vi "Main.vi"(7 "sweep rate, /min":dbl=0.2, 8 "sweep to:":dbl=4.0, 9 "sweep":T8(radio)=enum."2636a_smub") -> ()   [LabVIEW 2021] (continued)
                              }
                              frame True {
                                # "we are  measuring voltage on 2636A smua (2636A_smua_v)"
                                n1007 = local read "2614A addr"() -> (w1225:refnum<visa-resource-name>)
                                n1008 = call "SinglePointMeasurement.vi"("Measure"=Measure."Voltage", "Channel"=Channel."a", "VISA resource name 2"=w1225) -> ("Measuremet"=w1227:dbl)  [unwired: 3 in, 4 out]
                                n1009 = Build Array (concatenate)(w1230, w1227) -> (w1229:dbl[])
                              }
                            }
                            n1010 = property on="data" class="Arr (strict)"("Value"=w1223) -> ()  [unwired: 2 in, 2 out]
                          }
                          frame #25 {
                            # "check if current on\nKeithley 2636A smua\nis to be measured"
                            n1011 = local read "2636A smua meas i"() -> (w1231:bool)
                            n1012 = property on="data" class="Arr (strict)"() -> ("Value"=w1232:dbl[])  [unwired: 2 in, 2 out]
                            n1013 = case shown="True" w1231 {
                              tunnel: w1232 -> [w1234 w1237]
                              tunnel: [w1234 w1236] -> w1233
                              frame False {
                                # "we are not measuring current on 2636A smua (2636A_smua_i)"
                              }
                              frame True {
                                # "we are  measuring current on 2636A smua (2636A_smua_i)"
                                n1014 = stacked-sequence {
                                tunnel: [_ w1246] -> w1235
                                frame #0 {
                                n1015 = local read "auto\nrange A"() -> (w1241:bool)
                                n1016 = local read "2614A addr"() -> (w1244:refnum<visa-resource-name>)
                                n1017 = Select(t="smua.AUTORANGE_ON", s=w1241, f="smua.AUTORANGE_OFF") -> (s? t:f=w1239:string)
                                n1018 = Concatenate Strings("smua.measure.autorangei = ", w1239) -> (w1238:string)
                                n1019 = VISA Write(VISA resource name=w1244, write buffer=w1238) -> ()  [unwired: 1 in, 3 out]
                                }
                                frame #1 {
                                n1020 = local read "2614A addr"() -> (w1248:refnum<visa-resource-name>)
                                n1021 = call "SinglePointMeasurement.vi"("Measure"=Measure."Current", "Channel"=Channel."a", "VISA resource name 2"=w1248) -> ("Measuremet"=w1246:dbl)  [unwired: 3 in, 4 out]
                                }
                                }
                                n1022 = Build Array (concatenate)(w1237, w1235) -> (w1236:dbl[])
                              }
                            }
                            n1023 = property on="data" class="Arr (strict)"("Value"=w1233) -> ()  [unwired: 2 in, 2 out]
                          }
                          frame #26 {
                            # "check if voltage on\nKeithley 2636A smub\nis to be measured"
                            n1024 = local read "2636A smub meas v"() -> (w1249:bool)
                            n1025 = property on="data" class="Arr (strict)"() -> ("Value"=w1250:dbl[])  [unwired: 2 in, 2 out]
                            n1026 = case shown="True" w1249 {
                              tunnel: w1250 -> [w1252 w1258]
                              tunnel: [w1252 w1257] -> w1251
                              frame False {
                                # "we are not measuring voltage on 2636A smub (2636A_smub_v)"
                              }
                              frame True {
                                # "we are  measuring voltage on 2636A smub (2636A_smub_v)"
                                n1027 = local read "2614A addr"() -> (w1256:refnum<visa-resource-name>)
                                n1028 = call "SinglePointMeasurement.vi"("Measure"=Measure."Voltage", "Channel"=Channel."b", "VISA resource name 2"=w1256) -> ("Measuremet"=w1254:dbl)  [unwired: 3 in, 4 out]
                                n1029 = Build Array (concatenate)(w1258, w1254) -> (w1257:dbl[])
                              }
                            }
                            n1030 = property on="data" class="Arr (strict)"("Value"=w1251) -> ()  [unwired: 2 in, 2 out]
                          }
                          frame #27 {
                            # "check if current on\nKeithley 2636A smub\nis to be measured"
                            n1031 = local read "2636A smub meas i"() -> (w1259:bool)
                            n1032 = property on="data" class="Arr (strict)"() -> ("Value"=w1260:dbl[])  [unwired: 2 in, 2 out]
                            n1033 = case shown="True" w1259 {
                              tunnel: w1260 -> [w1262 w1265]
                              tunnel: [w1262 w1264] -> w1261
                              frame False {
                                # "we are not measuring current on 2636A smub (2636A_smub_i)"
                              }
                              frame True {
                                # "we are  measuring current on 2636A smub (2636A_smub_i)"
                                n1034 = stacked-sequence {
                                tunnel: [_ w1274] -> w1263
                                frame #0 {
                                n1035 = local read "auto\nrange B"() -> (w1269:bool)
                                n1036 = local read "2614A addr"() -> (w1272:refnum<visa-resource-name>)
                                n1037 = Select(t="smub.AUTORANGE_ON", s=w1269, f="smub.AUTORANGE_OFF") -> (s? t:f=w1267:string)
                                n1038 = Concatenate Strings("smub.measure.autorangei = ", w1267) -> (w1266:string)
                                n1039 = VISA Write(VISA resource name=w1272, write buffer=w1266) -> ()  [unwired: 1 in, 3 out]
                                }
                                frame #1 {
                                n1040 = local read "2614A addr"() -> (w1276:refnum<visa-resource-name>)
                                n1041 = call "SinglePointMeasurement.vi"("Measure"=Measure."Current", "Channel"=Channel."b", "VISA resource name 2"=w1276) -> ("Measuremet"=w1274:dbl)  [unwired: 3 in, 4 out]
                                }
                                }
                                n1042 = Build Array (concatenate)(w1265, w1263) -> (w1264:dbl[])
                              }
                            }
                            n1043 = property on="data" class="Arr (strict)"("Value"=w1261) -> ()  [unwired: 2 in, 2 out]
                          }
                          frame #28 {
                            # "check if time\nis to be measured"
                            n1044 = property on="data" class="Arr (strict)"() -> ("Value"=w1278:dbl[])  [unwired: 2 in, 2 out]
                            n1045 = local read "measure time"() -> (w1277:bool)
                            n1046 = case shown="True" w1277 {
                              tunnel: w1278 -> [w1280 w1283]
                              tunnel: [w1280 w1282] -> w1279
                              frame False {
                                # "we are not measuring time"
                              }
                              frame True {
                                # "seconds from the beginning of month"
                                # "we are  measuring time"
                                n1047 = Build Array (concatenate)(w1283, 0) -> (w1282:dbl[])
                              }
                            }
                            n1048 = property on="data" class="Arr (strict)"("Value"=w1279) -> ()  [unwired: 2 in, 2 out]
                          }
                          frame #29 {
                            n1049 = local read "MagnetField"() -> (w1284:bool)
                            n1050 = property on="data" class="Arr (strict)"() -> ("Value"=w1285:dbl[])  [unwired: 2 in, 2 out]
                            n1051 = case shown="True" w1284 {
                              tunnel: w1285 -> [w1287 w1292]
                              tunnel: [w1287 w1291] -> w1286
                              frame False {
                                # "we are not Measuring magnetic field on IPS120-0"
                              }
                              frame True {
                                # "Measure magnetic field on IPS120-0"
                                n1052 = local read "iPS_addr_sweep"() -> (w1290:refnum<visa-resource-name>)
                                n1053 = call "iPSread.vi"("iPSreadCtrl"=iPSreadCtrl."MagnetField", "VISA resource name"=w1290) -> ("number"=w1288:dbl)  [unwired: 6 in, 3 out]
                                n1054 = Build Array (concatenate)(w1292, w1288) -> (w1291:dbl[])
                              }
                            }
                            n1055 = property on="data" class="Arr (strict)"("Value"=w1286) -> ()  [unwired: 2 in, 2 out]
                          }
                          frame #30 {
                            n1056 = property on="data" class="Arr (strict)"() -> ("Value"=w1294:dbl[])  [unwired: 2 in, 2 out]
                            n1057 = property on="Magnet_T" class="Bool (strict)"() -> ("Value"=w1293:bool)  [unwired: 2 in, 2 out]
                            n1058 = case shown="True" w1293 {
                              tunnel: w1294 -> [w1296 w1301]
                              tunnel: [w1296 w1300] -> w1295
                              frame False {
                                # "we are not Measuring magnetic field on IPS120-0"
                              }
                              frame True {
                                # "Measure magnetic field on IPS120-0"
                                n1059 = local read "iPS_addr_sweep"() -> (w1299:refnum<visa-resource-name>)
                                n1060 = call "iPSread.vi"("iPSreadCtrl"=iPSreadCtrl."Magnet Temp", "VISA resource name"=w1299) -> ("number"=w1297:dbl)  [unwired: 6 in, 3 out]
                                n1061 = Build Array (concatenate)(w1301, w1297) -> (w1300:dbl[])
                              }
                            }
                            n1062 = property on="data" class="Arr (strict)"("Value"=w1295) -> ()  [unwired: 2 in, 2 out]
                          }
                          frame #31 {
                            n1063 = property on="PT1" class="Bool (strict)"() -> ("Value"=w1302:bool)  [unwired: 2 in, 2 out]
                            n1064 = property on="data" class="Arr (strict)"() -> ("Value"=w1303:dbl[])  [unwired: 2 in, 2 out]
                            n1065 = case shown="True" w1302 {
                              tunnel: w1303 -> [w1305 w1310]
                              tunnel: [w1305 w1309] -> w1304
                              frame False {
                                # "we are not Measuring magnetic field on IPS120-0"
                              }
                              frame True {
                                # "Measure magnetic field on IPS120-0"
                                n1066 = local read "iPS_addr_sweep"() -> (w1308:refnum<visa-resource-name>)
                                n1067 = call "iPSread.vi"("iPSreadCtrl"=iPSreadCtrl."Switch Heater Temp", "VISA resource name"=w1308) -> ("number"=w1306:dbl)  [unwired: 6 in, 3 out]
                                n1068 = Build Array (concatenate)(w1310, w1306) -> (w1309:dbl[])
                              }
                            }
                            n1069 = property on="data" class="Arr (strict)"("Value"=w1304) -> ()  [unwired: 2 in, 2 out]
                          }
                          frame #32 {
                            # "check if current \non 2461 SouceMeter\nis to be measured"
                            n1070 = property on="data" class="Arr (strict)"() -> ("Value"=w1312:dbl[])  [unwired: 2 in, 2 out]
                            n1071 = property on="MC_RuO2" class="Bool (strict)"() -> ("Value"=w1311:bool)  [unwired: 2 in, 2 out]
                            n1072 = case shown="True" w1311 {
                              tunnel: w1312 -> [w1314 w1319]
                              tunnel: [w1314 w1318] -> w1313
                              frame False {
                                # "we are not measuring 2461, voltage (2461_meas_v)"
                              }
                              frame True {
                                # "we are  measuring  Teslatron_iTC_Temp"
                                n1073 = property on="iPS_addr_sweep" class="VISAName"() -> ("Value"=w1315:refnum<visa-resource-name>)  [unwired: 2 in, 2 out]
                                n1074 = call "iTCread.vi"("VISA resource name"=w1315, "iTCreadCtrl"=iTCreadCtrl."Sample Temp") -> ("number"=w1316:dbl)  [unwired: 5 in, 3 out]
                                n1075 = Build Array (concatenate)(w1319, w1316) -> (w1318:dbl[])
                              }
                            }
                            n1076 = property on="data" class="Arr (strict)"("Value"=w1313) -> ()  [unwired: 2 in, 2 out]
                          }
                          frame #33 {
                            # "check if current \non 2461 SouceMeter\nis to be measured"
                            n1077 = property on="Still" class="Bool (strict)"() -> ("Value"=w1320:bool)  [unwired: 2 in, 2 out]
                            n1078 = property on="data" class="Arr (strict)"() -> ("Value"=w1321:dbl[])  [unwired: 2 in, 2 out]
                            n1079 = case shown="True" w1320 {
                              tunnel: w1321 -> [w1323 w1328]
                              tunnel: [w1323 w1327] -> w1322
                              frame False {
                                # "we are not measuring 2461, voltage (2461_meas_v)"
                              }
                              frame True {
                                # "we are  measuring  Teslatron_iTC_Temp"
                                n1080 = property on="iPS_addr_sweep" class="VISAName"() -> ("Value"=w1324:refnum<visa-resource-name>)  [unwired: 2 in, 2 out]
                                n1081 = call "iTCread.vi"("VISA resource name"=w1324, "iTCreadCtrl"=iTCreadCtrl."VTI Temp") -> ("number"=w1325:dbl)  [unwired: 5 in, 3 out]
                                n1082 = Build Array (concatenate)(w1328, w1325) -> (w1327:dbl[])
                              }
                            }
                            n1083 = property on="data" class="Arr (strict)"("Value"=w1322) -> ()  [unwired: 2 in, 2 out]
                          }
                          frame #34 {
                            # "check if current \non 2461 SouceMeter\nis to be measured"
                            n1084 = property on="Cold_Plate" class="Bool (strict)"() -> ("Value"=w1329:bool)  [unwired: 2 in, 2 out]
                            n1085 = property on="data" class="Arr (strict)"() -> ("Value"=w1330:dbl[])  [unwired: 2 in, 2 out]
                            n1086 = case shown="True" w1329 {
                              tunnel: w1330 -> [w1332 w1337]
                              tunnel: [w1332 w1336] -> w1331
                              frame False {
                                # "we are not measuring 2461, voltage (2461_meas_v)"
                              }
                              frame True {
                                # "we are  measuring  Teslatron_iTC_Temp"
                                n1087 = property on="iPS_addr_sweep" class="VISAName"() -> ("Value"=w1333:refnum<visa-resource-name>)  [unwired: 2 in, 2 out]
                                n1088 = call "iTCread.vi"("VISA resource name"=w1333, "iTCreadCtrl"=iTCreadCtrl."PT1 Temp") -> ("number"=w1334:dbl)  [unwired: 5 in, 3 out]
                                n1089 = Build Array (concatenate)(w1337, w1334) -> (w1336:dbl[])
                              }
                            }
                            n1090 = property on="data" class="Arr (strict)"("Value"=w1331) -> ()  [unwired: 2 in, 2 out]
                          }
                          frame #35 {
                            # "check if current \non 2461 SouceMeter\nis to be measured"
                            n1091 = property on="data" class="Arr (strict)"() -> ("Value"=w1339:dbl[])  [unwired: 2 in, 2 out]
                            n1092 = property on="PT2" class="Bool (strict)"() -> ("Value"=w1338:bool)  [unwired: 2 in, 2 out]
                            n1093 = case shown="True" w1338 {
                              tunnel: w1339 -> [w1341 w1346]
                              tunnel: [w1341 w1345] -> w1340
                              frame False {
                                # "we are not measuring 2461, voltage (2461_meas_v)"
                              }
                              frame True {
                                # "we are  measuring  Teslatron_iTC_Temp"
                                n1094 = property on="iPS_addr_sweep" class="VISAName"() -> ("Value"=w1342:refnum<visa-resource-name>)  [unwired: 2 in, 2 out]
                                n1095 = call "iTCread.vi"("VISA resource name"=w1342, "iTCreadCtrl"=iTCreadCtrl."PT2 Temp") -> ("number"=w1343:dbl)  [unwired: 5 in, 3 out]
                                n1096 = Build Array (concatenate)(w1346, w1343) -> (w1345:dbl[])
                              }
                            }
                            n1097 = property on="data" class="Arr (strict)"("Value"=w1340) -> ()  [unwired: 2 in, 2 out]
                          }
                          frame #36 {
                            # "check if current \non 2461 SouceMeter\nis to be measured"
                            n1098 = property on="data" class="Arr (strict)"() -> ("Value"=w1348:dbl[])  [unwired: 2 in, 2 out]
                            n1099 = property on="MC_Cernox" class="Bool (strict)"() -> ("Value"=w1347:bool)  [unwired: 2 in, 2 out]
                            n1100 = case shown="True" w1347 {
                              tunnel: w1348 -> [w1350 w1355]
                              tunnel: [w1350 w1354] -> w1349
                              frame False {
                                # "we are not measuring 2461, voltage (2461_meas_v)"
                              }
                              frame True {
                                # "we are  measuring  Teslatron_iTC_Temp"
                                n1101 = property on="iPS_addr_sweep" class="VISAName"() -> ("Value"=w1351:refnum<visa-resource-name>)  [unwired: 2 in, 2 out]
                                n1102 = call "iTCread.vi"("VISA resource name"=w1351, "iTCreadCtrl"=iTCreadCtrl."VTI Pressure") -> ("number"=w1352:dbl)  [unwired: 5 in, 3 out]
                                n1103 = Build Array (concatenate)(w1355, w1352) -> (w1354:dbl[])
                              }
                            }
                            n1104 = property on="data" class="Arr (strict)"("Value"=w1349) -> ()  [unwired: 2 in, 2 out]
                          }
                        }
                      }
                    }
                  }
                }
              }
            }
          }
          frame #4 {
            n1105 = Enqueue Element(queue=w1356, element="Idle") -> ()  [unwired: 2 in, 3 out]
            n1106 = Wait (ms)(milliseconds to wait="Refresh Time(ms)") -> ()  [unwired: 1 out]
          }
        }
      }
      frame "Line Traces" {
      }
      frame "Start Sweep" {
        w1362 = dbl[][] []  # emty array for data
        # "0 = SR830_1_ip\n1 = SR830_1_oop\n2 = SR830_2_ip\n3 = SR830_2_oop\n4 = SR830_3_ip\n5 = SR830_3_oop\n6 = SR830_4_ip \n7 = SR830_4_oop \n8 = SR830_5_ip \n9 = SR830_5_oop \n10= 2400_1_v \n11= 2400_1_i \n12 = 2400_2_v\n13 = 2400_2_i \n14 = 2400_3_v \n15 = 2400_3_i \n16 = 2182A_1_ch1 \n17 = 2182A_1_ch2 \n18 = 2182A_2_ch1 \n19 = 2182A_2_ch2\n20 = 2182A_3_ch1 \n21 = 2182A_3_ch2 \n22 = 2182A_4_ch1 \n23 = 2182A_4_ch2 \n24 = 2636A_smua_v \n25 = 2636A_smua_i \n26 = 2636A_smub_v \n27 = 2636A_smub_i \n28 = time\n29 = iPS_Field\n30 = iPS_Magnet_T\n31 = iPS__SH_T\n32 = iTC _sample_T\n33 = iTC _VTI_T\n34 = iTC _PT1_T\n35 = iTC _PT2_T\n36 = iTC _VTI_P\n37 = 2461_meas_v\n38= 2461_meas_i\n39= Step_Value\n40= HyperLoop_Step\n41= SuperHyper_Step\n42 = MFLI_V\n43 = MFLI_I"
        # "initial time in seconds\nfrom the beginning of month"
        n1107 = stacked-sequence {
          tunnel: [_ _ w2342 _ _ _] -> w1359
          frame #0 {
            n1108 = local read "2636A smua meas v"() -> (w1369:bool)
            n1109 = local read "2636A smub meas v"() -> (w1367:bool)
            n1110 = local read "2636A smub meas i"() -> (w1366:bool)
            n1111 = local read "2636A smua meas i"() -> (w1368:bool)
            n1112 = property on="sweep" class="RadioBtnsControl (strict)"() -> ("Value"=w1364:T8)  [unwired: 2 in, 2 out]
            n1113 = Compound Arithmetic op=OR(w1369, w1368, w1367, w1366) -> (w1365:bool)
            n1114 = case shown="\"AuxOut0\"" w1364 {
              frame "2400_1" {
                # "add label for the first column in the datafile"
                n1115 = stacked-sequence {
                  frame #0 {
                    n1116 = property on="data_caption" class="Str"("Value"="") -> ()  [unwired: 2 in, 2 out]
                    n1117 = property on="Figure_axis" class="Arr (strict)"("Value"=string[] [] ("Figure_axis_string")) -> ()  [unwired: 2 in, 2 out]
                  }
                  frame #1 {
                    w1372 = "V_sweep_2400_1" ("V_sweep")
                    n1118 = Concatenate Strings(w1372, "\t") -> (w1374:string)
                    n1119 = Build Array(w1372) -> (w1373:string[])
                    n1120 = property on="data_caption" class="Str"("Value"=w1374) -> ()  [unwired: 2 in, 2 out]
                    n1121 = property on="Figure_axis" class="Arr (strict)"("Value"=w1373) -> ()  [unwired: 2 in, 2 out]
                  }
                }
              }
              frame "2400_2" {
                n1122 = stacked-sequence {
                  frame #0 {
                    n1123 = property on="data_caption" class="Str"("Value"="") -> ()  [unwired: 2 in, 2 out]
                    n1124 = property on="Figure_axis" class="Arr (strict)"("Value"=string[] [] ("Figure_axis_string")) -> ()  [unwired: 2 in, 2 out]
                  }
                  frame #1 {
                    w1378 = "V_sweep_2400_2" ("V_sweep")
                    n1125 = Build Array(w1378) -> (w1379:string[])
                    n1126 = Concatenate Strings(w1378, "\t") -> (w1381:string)
                    n1127 = property on="Figure_axis" class="Arr (strict)"("Value"=w1379) -> ()  [unwired: 2 in, 2 out]
                    n1128 = property on="data_caption" class="Str"("Value"=w1381) -> ()  [unwired: 2 in, 2 out]
                  }
                }
              }
              frame "2400_3" {
                n1129 = stacked-sequence {
                  frame #0 {
                    n1130 = property on="data_caption" class="Str"("Value"="") -> ()  [unwired: 2 in, 2 out]
                    n1131 = property on="Figure_axis" class="Arr (strict)"("Value"=string[] [] ("Figure_axis_string")) -> ()  [unwired: 2 in, 2 out]
                  }
                  frame #1 {
                    w1384 = "V_sweep_2400_3" ("V_sweep")
                    n1132 = Concatenate Strings(w1384, "\t") -> (w1387:string)
                    n1133 = Build Array(w1384) -> (w1385:string[])
                    n1134 = property on="data_caption" class="Str"("Value"=w1387) -> ()  [unwired: 2 in, 2 out]
                    n1135 = property on="Figure_axis" class="Arr (strict)"("Value"=w1385) -> ()  [unwired: 2 in, 2 out]
                  }
                }
              }
              frame "2636a_smua" {
                n1136 = stacked-sequence {
                  frame #0 {
                    n1137 = property on="data_caption" class="Str"("Value"="") -> ()  [unwired: 2 in, 2 out]
                    n1138 = property on="Figure_axis" class="Arr (strict)"("Value"=string[] [] ("Figure_axis_string")) -> ()  [unwired: 2 in, 2 out]
                  }
                  frame #1 {
                    w1390 = "V_sweep_2614a_smua" ("V_sweep")
                    n1139 = Concatenate Strings(w1390, "\t") -> (w1393:string)
                    n1140 = Build Array(w1390) -> (w1391:string[])
                    n1141 = property on="data_caption" class="Str"("Value"=w1393) -> ()  [unwired: 2 in, 2 out]
                    n1142 = property on="Figure_axis" class="Arr (strict)"("Value"=w1391) -> ()  [unwired: 2 in, 2 out]
                  }
                }
              }
              frame "2636a_smub" {
                n1143 = stacked-sequence {
                  frame #0 {
                    n1144 = property on="data_caption" class="Str"("Value"="") -> ()  [unwired: 2 in, 2 out]
                    n1145 = property on="Figure_axis" class="Arr (strict)"("Value"=string[] [] ("Figure_axis_string")) -> ()  [unwired: 2 in, 2 out]
                  }
                  frame #1 {
                    w1396 = "V_sweep_2614a_smub" ("V_sweep")
                    n1146 = Build Array(w1396) -> (w1397:string[])
                    n1147 = Concatenate Strings(w1396, "\t") -> (w1399:string)
                    n1148 = property on="Figure_axis" class="Arr (strict)"("Value"=w1397) -> ()  [unwired: 2 in, 2 out]
                    n1149 = property on="data_caption" class="Str"("Value"=w1399) -> ()  [unwired: 2 in, 2 out]
                  }
                }
              }
              frame "time_sweep", Default {
                n1150 = stacked-sequence {
                  frame #0 {
                    n1151 = property on="data_caption" class="Str"("Value"="") -> ()  [unwired: 2 in, 2 out]
                    n1152 = property on="Figure_axis" class="Arr (strict)"("Value"=string[] [] ("Figure_axis_string")) -> ()  [unwired: 2 in, 2 out]
                  }
                  frame #1 {
                    w1402 = "time_sweep" ("V_sweep")
                    n1153 = Build Array(w1402) -> (w1403:string[])
                    n1154 = Concatenate Strings(w1402, "\t") -> (w1404:string)
                    n1155 = property on="Figure_axis" class="Arr (strict)"("Value"=w1403) -> ()  [unwired: 2 in, 2 out]
                    n1156 = property on="data_caption" class="Str"("Value"=w1404) -> ()  [unwired: 2 in, 2 out]
                  }
                }
              }
              frame "iPS" {
                n1157 = stacked-sequence {
                  frame #0 {
                    n1158 = property on="data_caption" class="Str"("Value"="") -> ()  [unwired: 2 in, 2 out]
                    n1159 = property on="Figure_axis" class="Arr (strict)"("Value"=string[] [] ("Figure_axis_string")) -> ()  [unwired: 2 in, 2 out]
                  }
                  frame #1 {
                    w1408 = "Teslatron_iPS_OutputField" ("V_sweep")
                    n1160 = Build Array(w1408) -> (w1409:string[])
                    n1161 = Concatenate Strings(w1408, "\t") -> (w1411:string)
                    n1162 = property on="Figure_axis" class="Arr (strict)"("Value"=w1409) -> ()  [unwired: 2 in, 2 out]
                    n1163 = property on="data_caption" class="Str"("Value"=w1411) -> ()  [unwired: 2 in, 2 out]
                  }
                }
              }
              frame "iTC" {
                n1164 = stacked-sequence {
                  frame #0 {
                    n1165 = property on="data_caption" class="Str"("Value"="") -> ()  [unwired: 2 in, 2 out]
                    n1166 = property on="Figure_axis" class="Arr (strict)"("Value"=string[] ["", "SR830_1_ip", "SR830_1_oop", "SR830_2_ip", "SR830_2_oop", "2461_meas_v", "2461_meas_i", "2636A_smua_v", "2636A_smua_i", "formula"] ("Figure_axis")) -> ()  [unwired: 2 in, 2 out]
                  }
                  frame #1 {
                    w1416 = "Teslatron_iTC_Temp"
                    n1167 = Build Array(w1416) -> (w1415:string[])
                    n1168 = Concatenate Strings(w1416, "\t") -> (w1414:string)
                    n1169 = property on="data_caption" class="Str"("Value"=w1414) -> ()  [unwired: 2 in, 2 out]
                    n1170 = property on="Figure_axis" class="Arr (strict)"("Value"=w1415) -> ()  [unwired: 2 in, 2 out]
                  }
                }
              }
              frame "2461" {
                n1171 = stacked-sequence {
                  frame #0 {
                    n1172 = property on="data_caption" class="Str"("Value"="") -> ()  [unwired: 2 in, 2 out]
                    n1173 = property on="Figure_axis" class="Arr (strict)"("Value"=string[] ["", "SR830_1_ip", "SR830_1_oop", "SR830_2_ip", "SR830_2_oop", "2461_meas_v", "2461_meas_i", "2636A_smua_v", "2636A_smua_i", "formula"] ("Figure_axis")) -> ()  [unwired: 2 in, 2 out]
                  }
                  frame #1 {
                    w1422 = "I_sweep_2461"
                    n1174 = Build Array(w1422) -> (w1421:string[])
                    n1175 = Concatenate Strings(w1422, "\t") -> (w1420:string)
                    n1176 = property on="data_caption" class="Str"("Value"=w1420) -> ()  [unwired: 2 in, 2 out]
                    n1177 = property on="Figure_axis" class="Arr (strict)"("Value"=w1421) -> ()  [unwired: 2 in, 2 out]
                  }
                }
              }
              frame "AuxOut0" {
                n1178 = stacked-sequence {
                  frame #0 {
                    n1179 = property on="data_caption" class="Str"("Value"="") -> ()  [unwired: 2 in, 2 out]
                    n1180 = property on="Figure_axis" class="Arr (strict)"("Value"=string[] ["", "SR830_1_ip", "SR830_1_oop", "SR830_2_ip", "SR830_2_oop", "2461_meas_v", "2461_meas_i", "2636A_smua_v", "2636A_smua_i", "formula"] ("Figure_axis")) -> ()  [unwired: 2 in, 2 out]
                  }
                  frame #1 {
                    w1428 = "V_Sweep_AuxOut0"
                    n1181 = Build Array(w1428) -> (w1427:string[])
                    n1182 = Concatenate Strings(w1428, "\t") -> (w1426:string)
                    n1183 = property on="data_caption" class="Str"("Value"=w1426) -> ()  [unwired: 2 in, 2 out]
                    n1184 = property on="Figure_axis" class="Arr (strict)"("Value"=w1427) -> ()  [unwired: 2 in, 2 out]
                  }
                }
              }
            }
            n1185 = case shown="True" w1365 {
              frame False {
              }
              frame True {
                # "opens session for 2636a system sourcemeter"
                n1186 = local read "2614A addr"() -> (w1430:refnum<visa-resource-name>)
                n1187 = VISA Open(VISA resource name=w1430) -> ()  [unwired: 4 in, 2 out]
              }
            }
          }
          frame #1 {
            # "0 = SR830_1_ip\n1 = SR830_1_oop\n2 = SR830_2_ip\n3 = SR830_2_oop\n4 = SR830_3_ip\n5 = SR830_3_oop\n6 = SR830_4_ip \n7 = SR830_4_oop \n8 = SR830_5_ip \n9 = SR830_5_oop \n10= 2400_1_v \n11= 2400_1_i \n12 = 2400_2_v\n13 = 2400_2_i \n14 = 2400_3_v \n15 = 2400_3_i \n16 = 2182A_1_ch1 \n17 = 2182A_1_ch2 \n18 = 2182A_2_ch1 \n19 = 2182A_2_ch2\n20 = 2182A_3_ch1 \n21 = 2182A_3_ch2 \n22 = 2182A_4_ch1 \n23 = 2182A_4_ch2 \n24 = 2636A_smua_v \n25 = 2636A_smua_i \n26 = 2636A_smub_v \n27 = 2636A_smub_i \n28 = time\n29 = iPS_Field\n30 = iPS_Magnet_T\n31 = iPS__SH_T\n32 = iTC _sample_T\n33 = iTC _VTI_T\n34 = iTC _PT1_T\n35 = iTC _PT2_T\n36 = iTC _VTI_P\n37 = 2461_meas_v\n38= 2461_meas_i\n39= Step_Value\n40= HyperLoop_Step\n41= SuperHyper_Step\n42 = MFLI_V\n43 = MFLI_I"
            # "this part constructs the first (text) line for the data file with names of all measured variables,\nalso constructs a text array contaning names of all measured variable for the \"ring\" (so parameter can be selected and plotted)"
            n1188 = stacked-sequence {
              tunnel: [w1431 _ _ _ _ _ _ _ _ _ _ _ _ _ _ _ _ _ _ _ _ _ _ _ _ _ _ _ _ _ _ _ _ _ _ _ _ _ _ _ _ _ _ _ _ _ _ _ _ _ _ _ _ _ _ _ _ _ _] -> _
              frame #0 {
                # "SR830 1 in phase (SR830_1_ip)"
                n1189 = local read "SR830 1 ip"() -> (w1436:bool)
                n1190 = property on="Figure_axis" class="Arr (strict)"() -> ("Value"=w1433:string[])  [unwired: 2 in, 2 out]
                n1191 = property on="data_caption" class="Str"() -> ("Value"=w1435:string)  [unwired: 2 in, 2 out]
                n1192 = case shown="True" w1436 {
                  tunnel: w1435 -> [w1438 w1444]
                  tunnel: [w1438 w1443] -> w1434
                  tunnel: w1433 -> [w1437 w1441]
                  tunnel: [w1437 w1439] -> w1432
                  frame False {
                    # "not measure SR830 1 in phase signal (SR830_1_ip)"
                  }
                  frame True {
                    w1440 = "SR830_1_ip"
                    # "measure SR830 1 in phase signal (SR830_1_ip)"
                    n1193 = local read "SR830 1 addr"() -> (w1445:u8)
                    n1194 = Number To Decimal String(number=w1445) -> (decimal integer string=w1446:string)  [unwired: 1 in]
                    n1195 = GPIB Clear(3:w1446) -> ()  [unwired: 1 in, 2 out]
                    n1196 = Build Array (concatenate)(w1441, w1440) -> (w1439:string[])
                    n1197 = Concatenate Strings(w1444, w1440, "\t") -> (w1443:string)
                  }
                }
                n1198 = property on="Figure_axis" class="Arr (strict)"("Value"=w1432) -> ()  [unwired: 2 in, 2 out]
                n1199 = property on="data_caption" class="Str"("Value"=w1434) -> (error out=w1431:errorcluster)  [unwired: 2 in, 1 out]
              }
              frame #1 {
                # "SR830 1 out of phase (SR830_1_oop)"
                n1200 = local read "SR830 1 oop"() -> (w1451:bool)
                n1201 = property on="Figure_axis" class="Arr (strict)"() -> ("Value"=w1448:string[])  [unwired: 2 in, 2 out]
                n1202 = property on="data_caption" class="Str"() -> ("Value"=w1450:string)  [unwired: 2 in, 2 out]
                n1203 = case shown="False" w1451 {
                  tunnel: w1450 -> [w1453 w1459]
                  tunnel: [w1453 w1458] -> w1449
                  tunnel: w1448 -> [w1452 w1456]
                  tunnel: [w1452 w1454] -> w1447
                  frame False {
                    # "not measure SR830 1 out of phase signal (SR830_1_oop)"
                  }
                  frame True {
                    w1455 = "SR830_1_oop"
                    # "measure SR830 1 out of phase signal (SR830_1_oop)"
                    n1204 = local read "SR830 1 addr"() -> (w1460:u8)
                    n1205 = Number To Decimal String(number=w1460) -> (decimal integer string=w1461:string)  [unwired: 1 in]
                    n1206 = GPIB Clear(3:w1461) -> ()  [unwired: 1 in, 2 out]
                    n1207 = Build Array (concatenate)(w1456, w1455) -> (w1454:string[])
                    n1208 = Concatenate Strings(w1459, w1455, "\t") -> (w1458:string)
                  }
                }
                n1209 = property on="Figure_axis" class="Arr (strict)"("Value"=w1447) -> ()  [unwired: 2 in, 2 out]
                n1210 = property on="data_caption" class="Str"("Value"=w1449) -> ()  [unwired: 2 in, 2 out]
              }
              frame #2 {
                # "SR830 2 in phase (SR830_2_ip)"
                n1211 = local read "SR830 2 ip"() -> (w1466:bool)
                n1212 = property on="Figure_axis" class="Arr (strict)"() -> ("Value"=w1463:string[])  [unwired: 2 in, 2 out]
                n1213 = property on="data_caption" class="Str"() -> ("Value"=w1465:string)  [unwired: 2 in, 2 out]
                n1214 = case shown="False" w1466 {
                  tunnel: w1465 -> [w1468 w1474]
                  tunnel: [w1468 w1473] -> w1464
                  tunnel: w1463 -> [w1467 w1471]
                  tunnel: [w1467 w1469] -> w1462
                  frame False {
                    # "not measure SR830 2 in phase signal (SR830_2_ip)"
                  }
                  frame True {
                    w1470 = "SR830_2_ip"
                    # "measure SR830 2 in phase signal (SR830_2_ip)"
                    n1215 = local read "SR830 2 addr"() -> (w1475:u8)
                    n1216 = Number To Decimal String(number=w1475) -> (decimal integer string=w1476:string)  [unwired: 1 in]
                    n1217 = GPIB Clear(3:w1476) -> ()  [unwired: 1 in, 2 out]
                    n1218 = Build Array (concatenate)(w1471, w1470) -> (w1469:string[])
                    n1219 = Concatenate Strings(w1474, w1470, "\t") -> (w1473:string)
                  }
                }
                n1220 = property on="Figure_axis" class="Arr (strict)"("Value"=w1462) -> ()  [unwired: 2 in, 2 out]
                n1221 = property on="data_caption" class="Str"("Value"=w1464) -> ()  [unwired: 2 in, 2 out]
              }
              frame #3 {
                # "SR830 2 out of phase (SR830_2_oop)"
                n1222 = local read "SR830 2 oop"() -> (w1481:bool)
                n1223 = property on="Figure_axis" class="Arr (strict)"() -> ("Value"=w1478:string[])  [unwired: 2 in, 2 out]
                n1224 = property on="data_caption" class="Str"() -> ("Value"=w1480:string)  [unwired: 2 in, 2 out]
                n1225 = case shown="False" w1481 {
                  tunnel: w1480 -> [w1483 w1489]
                  tunnel: [w1483 w1488] -> w1479
                  tunnel: w1478 -> [w1482 w1486]
                  tunnel: [w1482 w1484] -> w1477
                  frame False {
                    # "not measure SR830 2 out of phase signal (SR830_2_oop)"
                  }
                  frame True {
                    w1485 = "SR830_2_oop"
                    # "measure SR830 2 out of phase signal (SR830_2_oop)"
                    n1226 = local read "SR830 2 addr"() -> (w1490:u8)
                    n1227 = Number To Decimal String(number=w1490) -> (decimal integer string=w1491:string)  [unwired: 1 in]
                    n1228 = GPIB Clear(3:w1491) -> ()  [unwired: 1 in, 2 out]
                    n1229 = Build Array (concatenate)(w1486, w1485) -> (w1484:string[])
                    n1230 = Concatenate Strings(w1489, w1485, "\t") -> (w1488:string)
                  }
                }
                n1231 = property on="Figure_axis" class="Arr (strict)"("Value"=w1477) -> ()  [unwired: 2 in, 2 out]
                n1232 = property on="data_caption" class="Str"("Value"=w1479) -> ()  [unwired: 2 in, 2 out]
              }
              frame #4 {
                # "SR830 3 in phase (SR830_3_ip)"
                n1233 = local read "SR830 3 ip"() -> (w1496:bool)
                n1234 = property on="Figure_axis" class="Arr (strict)"() -> ("Value"=w1493:string[])  [unwired: 2 in, 2 out]
                n1235 = property on="data_caption" class="Str"() -> ("Value"=w1495:string)  [unwired: 2 in, 2 out]
                n1236 = case shown="False" w1496 {
                  tunnel: w1495 -> [w1498 w1504]
                  tunnel: [w1498 w1503] -> w1494
                  tunnel: w1493 -> [w1497 w1501]
                  tunnel: [w1497 w1499] -> w1492
                  frame False {
                    # "not measure SR830 3 in phase signal (SR830_3_ip)"
                  }
                  frame True {
                    w1500 = "SR830_3_ip"
                    # "measure SR830 3 in phase signal (SR830_3_ip)"
                    n1237 = local read "SR830 3 addr"() -> (w1505:u8)
                    n1238 = Number To Decimal String(number=w1505) -> (decimal integer string=w1506:string)  [unwired: 1 in]
                    n1239 = GPIB Clear(3:w1506) -> ()  [unwired: 1 in, 2 out]
                    n1240 = Build Array (concatenate)(w1501, w1500) -> (w1499:string[])
                    n1241 = Concatenate Strings(w1504, w1500, "\t") -> (w1503:string)
                  }
                }
                n1242 = property on="Figure_axis" class="Arr (strict)"("Value"=w1492) -> ()  [unwired: 2 in, 2 out]
                n1243 = property on="data_caption" class="Str"("Value"=w1494) -> ()  [unwired: 2 in, 2 out]
              }
              frame #5 {
                # "SR830 3 out of phase (SR830_3_oop)"
                n1244 = local read "SR830 3 oop"() -> (w1511:bool)
                n1245 = property on="Figure_axis" class="Arr (strict)"() -> ("Value"=w1508:string[])  [unwired: 2 in, 2 out]
                n1246 = property on="data_caption" class="Str"() -> ("Value"=w1510:string)  [unwired: 2 in, 2 out]
                n1247 = case shown="False" w1511 {
                  tunnel: w1510 -> [w1513 w1519]
                  tunnel: [w1513 w1518] -> w1509
                  tunnel: w1508 -> [w1512 w1516]
                  tunnel: [w1512 w1514] -> w1507
                  frame False {
                    # "not measure SR830 3 out of phase signal (SR830_3_oop)"
                  }
                  frame True {
                    w1515 = "SR830_3_oop"
                    # "measure SR830 3 out phase signal (SR830_3_oop)"
                    n1248 = local read "SR830 3 addr"() -> (w1520:u8)
                    n1249 = Number To Decimal String(number=w1520) -> (decimal integer string=w1521:string)  [unwired: 1 in]
                    n1250 = GPIB Clear(3:w1521) -> ()  [unwired: 1 in, 2 out]
                    n1251 = Build Array (concatenate)(w1516, w1515) -> (w1514:string[])
                    n1252 = Concatenate Strings(w1519, w1515, "\t") -> (w1518:string)
                  }
                }
                n1253 = property on="Figure_axis" class="Arr (strict)"("Value"=w1507) -> ()  [unwired: 2 in, 2 out]
                n1254 = property on="data_caption" class="Str"("Value"=w1509) -> ()  [unwired: 2 in, 2 out]
              }
              frame #6 {
                # "SR830 4 in phase (SR830_4_ip)"
                n1255 = local read "SR830 4 ip"() -> (w1526:bool)
                n1256 = property on="Figure_axis" class="Arr (strict)"() -> ("Value"=w1523:string[])  [unwired: 2 in, 2 out]
                n1257 = property on="data_caption" class="Str"() -> ("Value"=w1525:string)  [unwired: 2 in, 2 out]
                n1258 = case shown="False" w1526 {
                  tunnel: w1525 -> [w1528 w1534]
                  tunnel: [w1528 w1533] -> w1524
                  tunnel: w1523 -> [w1527 w1531]
                  tunnel: [w1527 w1529] -> w1522
                  frame False {
                    # "not measure SR830 4 in phase signal (SR830_4_ip)"
                  }
                  frame True {
                    w1530 = "SR830_4_ip"
                    # "measure SR830 4 in phase signal (SR830_4_ip)"
                    n1259 = local read "SR830 4 addr"() -> (w1535:u8)
                    n1260 = Number To Decimal String(number=w1535) -> (decimal integer string=w1536:string)  [unwired: 1 in]
                    n1261 = GPIB Clear(3:w1536) -> ()  [unwired: 1 in, 2 out]
                    n1262 = Build Array (concatenate)(w1531, w1530) -> (w1529:string[])
                    n1263 = Concatenate Strings(w1534, w1530, "\t") -> (w1533:string)
                  }
                }
                n1264 = property on="Figure_axis" class="Arr (strict)"("Value"=w1522) -> ()  [unwired: 2 in, 2 out]
                n1265 = property on="data_caption" class="Str"("Value"=w1524) -> ()  [unwired: 2 in, 2 out]
              }
              frame #7 {
                # "SR830 4 out of phase (SR830_4_oop)"
                n1266 = local read "SR830 4 oop"() -> (w1541:bool)
                n1267 = property on="Figure_axis" class="Arr (strict)"() -> ("Value"=w1538:string[])  [unwired: 2 in, 2 out]
                n1268 = property on="data_caption" class="Str"() -> ("Value"=w1540:string)  [unwired: 2 in, 2 out]
                n1269 = case shown="False" w1541 {
                  tunnel: w1540 -> [w1543 w1549]
                  tunnel: [w1543 w1548] -> w1539
                  tunnel: w1538 -> [w1542 w1546]
                  tunnel: [w1542 w1544] -> w1537
                  frame False {
                    # "not measure SR830 4 out of phase signal (SR830_4_oop)"
                  }
                  frame True {
                    w1545 = "SR830_4_oop"
                    # "measure SR830 4 out of phase signal (SR830_4_oop)"
                    n1270 = local read "SR830 4 addr"() -> (w1550:u8)
                    n1271 = Number To Decimal String(number=w1550) -> (decimal integer string=w1551:string)  [unwired: 1 in]
                    n1272 = GPIB Clear(3:w1551) -> ()  [unwired: 1 in, 2 out]
                    n1273 = Build Array (concatenate)(w1546, w1545) -> (w1544:string[])
                    n1274 = Concatenate Strings(w1549, w1545, "\t") -> (w1548:string)
                  }
                }
                n1275 = property on="Figure_axis" class="Arr (strict)"("Value"=w1537) -> ()  [unwired: 2 in, 2 out]
                n1276 = property on="data_caption" class="Str"("Value"=w1539) -> ()  [unwired: 2 in, 2 out]
              }
              frame #8 {
                # "SR830 5 in phase (SR830_5_ip)"
                n1277 = local read "SR830 5 ip"() -> (w1556:bool)
                n1278 = property on="Figure_axis" class="Arr (strict)"() -> ("Value"=w1553:string[])  [unwired: 2 in, 2 out]
                n1279 = property on="data_caption" class="Str"() -> ("Value"=w1555:string)  [unwired: 2 in, 2 out]
                n1280 = case shown="True" w1556 {
                  tunnel: w1555 -> [w1558 w1564]
                  tunnel: [w1558 w1563] -> w1554
                  tunnel: w1553 -> [w1557 w1561]
                  tunnel: [w1557 w1559] -> w1552
                  frame False {
                    # "not measure SR830 5 in phase signal (SR830_5_ip)"
                  }
                  frame True {
                    w1560 = "SR830_5_ip"
                    # "measure SR830 5 in phase signal (SR830_5_ip)"
                    n1281 = local read "SR830 5 addr"() -> (w1565:u8)
                    n1282 = Number To Decimal String(number=w1565) -> (decimal integer string=w1566:string)  [unwired: 1 in]
                    n1283 = GPIB Clear(3:w1566) -> ()  [unwired: 1 in, 2 out]
                    n1284 = Build Array (concatenate)(w1561, w1560) -> (w1559:string[])
                    n1285 = Concatenate Strings(w1564, w1560, "\t") -> (w1563:string)
                  }
                }
                n1286 = property on="Figure_axis" class="Arr (strict)"("Value"=w1552) -> ()  [unwired: 2 in, 2 out]
                n1287 = property on="data_caption" class="Str"("Value"=w1554) -> ()  [unwired: 2 in, 2 out]
              }
              frame #9 {
                # "SR830 5 out of phase (SR830_5_oop)"
                n1288 = local read "SR830 5 oop"() -> (w1571:bool)
                n1289 = property on="Figure_axis" class="Arr (strict)"() -> ("Value"=w1568:string[])  [unwired: 2 in, 2 out]
                n1290 = property on="data_caption" class="Str"() -> ("Value"=w1570:string)  [unwired: 2 in, 2 out]
                n1291 = case shown="True" w1571 {
                  tunnel: w1570 -> [w1573 w1579]
                  tunnel: [w1573 w1578] -> w1569
                  tunnel: w1568 -> [w1572 w1576]
                  tunnel: [w1572 w1574] -> w1567
                  frame False {
                    # "not measure SR830 5 out of phase signal (SR830_5_oop)"
                  }
                  frame True {
                    w1575 = "SR830_5_oop"
                    # "measure SR830 5 out of phase signal (SR830_5_oop)"
                    n1292 = local read "SR830 5 addr"() -> (w1580:u8)
                    n1293 = Number To Decimal String(number=w1580) -> (decimal integer string=w1581:string)  [unwired: 1 in]
                    n1294 = GPIB Clear(3:w1581) -> ()  [unwired: 1 in, 2 out]
                    n1295 = Build Array (concatenate)(w1576, w1575) -> (w1574:string[])
                    n1296 = Concatenate Strings(w1579, w1575, "\t") -> (w1578:string)
                  }
                }
                n1297 = property on="Figure_axis" class="Arr (strict)"("Value"=w1567) -> ()  [unwired: 2 in, 2 out]
                n1298 = property on="data_caption" class="Str"("Value"=w1569) -> ()  [unwired: 2 in, 2 out]
              }
              frame #10 {
                # "2400 1 voltage measure (2400_1_v)"
                n1299 = local read "2400 1 meas v"() -> (w1586:bool)
                n1300 = property on="Figure_axis" class="Arr (strict)"() -> ("Value"=w1583:string[])  [unwired: 2 in, 2 out]
                n1301 = property on="data_caption" class="Str"() -> ("Value"=w1585:string)  [unwired: 2 in, 2 out]
                n1302 = case shown="False" w1586 {
                  tunnel: w1585 -> [w1588 w1594]
                  tunnel: [w1588 w1593] -> w1584
                  tunnel: w1583 -> [w1587 w1591]
                  tunnel: [w1587 w1589] -> w1582
                  frame False {
                    # "not measure 2400 1 voltage (2400_1_v)"
                  }
                  frame True {
                    w1590 = "2400_1_v"
                    # "measure 2400 1 voltage (2400_1_v)"
                    n1303 = local read "2400 1 addr"() -> (w1595:u8)
                    n1304 = Number To Decimal String(number=w1595) -> (decimal integer string=w1596:string)  [unwired: 1 in]
                    n1305 = GPIB Clear(3:w1596) -> ()  [unwired: 1 in, 2 out]
                    n1306 = Build Array (concatenate)(w1591, w1590) -> (w1589:string[])
                    n1307 = Concatenate Strings(w1594, w1590, "\t") -> (w1593:string)
                  }
                }
                n1308 = property on="Figure_axis" class="Arr (strict)"("Value"=w1582) -> ()  [unwired: 2 in, 2 out]
                n1309 = property on="data_caption" class="Str"("Value"=w1584) -> ()  [unwired: 2 in, 2 out]
              }
              frame #11 {
                # "2400 1 current measure (2400_1_i)"
                n1310 = local read "2400 1 meas i"() -> (w1601:bool)
                n1311 = property on="Figure_axis" class="Arr (strict)"() -> ("Value"=w1598:string[])  [unwired: 2 in, 2 out]
                n1312 = property on="data_caption" class="Str"() -> ("Value"=w1600:string)  [unwired: 2 in, 2 out]
                n1313 = case shown="False" w1601 {
                  tunnel: w1600 -> [w1603 w1609]
                  tunnel: [w1603 w1608] -> w1599
                  tunnel: w1598 -> [w1602 w1606]
                  tunnel: [w1602 w1604] -> w1597
                  frame False {
                    # "not measure 2400 1 current (2400_1_i)"
                  }
                  frame True {
                    w1605 = "2400_1_i"
                    # "measure 2400 1 current (2400_1_i)"
                    n1314 = local read "2400 1 addr"() -> (w1610:u8)
                    n1315 = Number To Decimal String(number=w1610) -> (decimal integer string=w1611:string)  [unwired: 1 in]
                    n1316 = GPIB Clear(3:w1611) -> ()  [unwired: 1 in, 2 out]
                    n1317 = Build Array (concatenate)(w1606, w1605) -> (w1604:string[])
                    n1318 = Concatenate Strings(w1609, w1605, "\t") -> (w1608:string)
                  }
                }
                n1319 = property on="Figure_axis" class="Arr (strict)"("Value"=w1597) -> ()  [unwired: 2 in, 2 out]
                n1320 = property on="data_caption" class="Str"("Value"=w1599) -> ()  [unwired: 2 in, 2 out]
              }
              frame #12 {
                # "2400 2 voltage measure (2400_2_v)"
                n1321 = local read "2400 2 meas v"() -> (w1616:bool)
                n1322 = property on="Figure_axis" class="Arr (strict)"() -> ("Value"=w1613:string[])  [unwired: 2 in, 2 out]
                n1323 = property on="data_caption" class="Str"() -> ("Value"=w1615:string)  [unwired: 2 in, 2 out]
                n1324 = case shown="False" w1616 {
                  tunnel: w1615 -> [w1618 w1624]
                  tunnel: [w1618 w1623] -> w1614
                  tunnel: w1613 -> [w1617 w1621]
                  tunnel: [w1617 w1619] -> w1612
                  frame False {
                    # "not measure 2400 2 voltage (2400_2_v)"
                  }
                  frame True {
                    w1620 = "2400_2_v"
                    # "measure 2400 2 voltage (2400_2_v)"
                    n1325 = local read "2400 2 addr"() -> (w1625:u8)
                    n1326 = Number To Decimal String(number=w1625) -> (decimal integer string=w1626:string)  [unwired: 1 in]
                    n1327 = GPIB Clear(3:w1626) -> ()  [unwired: 1 in, 2 out]
                    n1328 = Build Array (concatenate)(w1621, w1620) -> (w1619:string[])
                    n1329 = Concatenate Strings(w1624, w1620, "\t") -> (w1623:string)
                  }
                }
                n1330 = property on="Figure_axis" class="Arr (strict)"("Value"=w1612) -> ()  [unwired: 2 in, 2 out]
                n1331 = property on="data_caption" class="Str"("Value"=w1614) -> ()  [unwired: 2 in, 2 out]
              }
              frame #13 {
                # "2400 2 current measure (2400_2_i)"
                n1332 = local read "2400 2 meas i"() -> (w1631:bool)
                n1333 = property on="Figure_axis" class="Arr (strict)"() -> ("Value"=w1628:string[])  [unwired: 2 in, 2 out]
                n1334 = property on="data_caption" class="Str"() -> ("Value"=w1630:string)  [unwired: 2 in, 2 out]
                n1335 = case shown="False" w1631 {
                  tunnel: w1630 -> [w1633 w1639]
                  tunnel: [w1633 w1638] -> w1629
                  tunnel: w1628 -> [w1632 w1636]
                  tunnel: [w1632 w1634] -> w1627
                  frame False {
                    # "not measure 2400 2 current (2400_2_i)"
                  }
                  frame True {
                    w1635 = "2400_2_i"
                    # "measure 2400 2 current (2400_2_i)"
                    n1336 = local read "2400 2 addr"() -> (w1640:u8)
                    n1337 = Number To Decimal String(number=w1640) -> (decimal integer string=w1641:string)  [unwired: 1 in]
                    n1338 = GPIB Clear(3:w1641) -> ()  [unwired: 1 in, 2 out]
                    n1339 = Build Array (concatenate)(w1636, w1635) -> (w1634:string[])
                    n1340 = Concatenate Strings(w1639, w1635, "\t") -> (w1638:string)
                  }
                }
                n1341 = property on="Figure_axis" class="Arr (strict)"("Value"=w1627) -> ()  [unwired: 2 in, 2 out]
                n1342 = property on="data_caption" class="Str"("Value"=w1629) -> ()  [unwired: 2 in, 2 out]
              }
              frame #14 {
                # "2400 3 voltage measure (2400_3_v)"
                n1343 = local read "2400 3 meas v"() -> (w1646:bool)
                n1344 = property on="Figure_axis" class="Arr (strict)"() -> ("Value"=w1643:string[])  [unwired: 2 in, 2 out]
                n1345 = property on="data_caption" class="Str"() -> ("Value"=w1645:string)  [unwired: 2 in, 2 out]
                n1346 = case shown="False" w1646 {
                  tunnel: w1645 -> [w1648 w1654]
                  tunnel: [w1648 w1653] -> w1644
                  tunnel: w1643 -> [w1647 w1651]
                  tunnel: [w1647 w1649] -> w1642
                  frame False {
                    # "not measure 2400 3 voltage (2400_3_v)"
                  }
                  frame True {
                    w1650 = "2400_3_v"
                    # "measure 2400 3 voltage (2400_3_v)"
                    n1347 = local read "2400 3 addr"() -> (w1655:u8)
                    n1348 = Number To Decimal String(number=w1655) -> (decimal integer string=w1656:string)  [unwired: 1 in]
                    n1349 = GPIB Clear(3:w1656) -> ()  [unwired: 1 in, 2 out]
                    n1350 = Build Array (concatenate)(w1651, w1650) -> (w1649:string[])
                    n1351 = Concatenate Strings(w1654, w1650, "\t") -> (w1653:string)
                  }
                }
                n1352 = property on="Figure_axis" class="Arr (strict)"("Value"=w1642) -> ()  [unwired: 2 in, 2 out]
                n1353 = property on="data_caption" class="Str"("Value"=w1644) -> ()  [unwired: 2 in, 2 out]
              }
              frame #15 {
                # "2400 3 current measure (2400_3_i)"
                n1354 = local read "2400 3 meas i"() -> (w1661:bool)
                n1355 = property on="Figure_axis" class="Arr (strict)"() -> ("Value"=w1658:string[])  [unwired: 2 in, 2 out]
                n1356 = property on="data_caption" class="Str"() -> ("Value"=w1660:string)  [unwired: 2 in, 2 out]
                n1357 = case shown="True" w1661 {
                  tunnel: w1660 -> [w1663 w1669]
                  tunnel: [w1663 w1668] -> w1659
                  tunnel: w1658 -> [w1662 w1666]
                  tunnel: [w1662 w1664] -> w1657
                  frame False {
                    # "not measure 2400 3 current (2400_3_i)"
                  }
                  frame True {
                    w1665 = "2400_3_i"
                    # "measure 2400 3 current (2400_3_i)"
                    n1358 = local read "2400 3 addr"() -> (w1670:u8)
                    n1359 = Number To Decimal String(number=w1670) -> (decimal integer string=w1671:string)  [unwired: 1 in]
                    n1360 = GPIB Clear(3:w1671) -> ()  [unwired: 1 in, 2 out]
                    n1361 = Build Array (concatenate)(w1666, w1665) -> (w1664:string[])
                    n1362 = Concatenate Strings(w1669, w1665, "\t") -> (w1668:string)
                  }
                }
                n1363 = property on="Figure_axis" class="Arr (strict)"("Value"=w1657) -> ()  [unwired: 2 in, 2 out]
                n1364 = property on="data_caption" class="Str"("Value"=w1659) -> ()  [unwired: 2 in, 2 out]
              }
              frame #16 {
                # "2182A 1 channel 1 measure (2182A_1_ch1)"
                n1365 = local read "2182A 1 ch1"() -> (w1676:bool)
                n1366 = property on="Figure_axis" class="Arr (strict)"() -> ("Value"=w1673:string[])  [unwired: 2 in, 2 out]
                n1367 = property on="data_caption" class="Str"() -> ("Value"=w1675:string)  [unwired: 2 in, 2 out]
                n1368 = case shown="False" w1676 {
                  tunnel: w1675 -> [w1678 w1684]
                  tunnel: [w1678 w1683] -> w1674
                  tunnel: w1673 -> [w1677 w1681]
                  tunnel: [w1677 w1679] -> w1672
                  frame False {
                    # "not measure 2182A 1 channel 1 (2182A_1_ch1)"
                  }
                  frame True {
                    w1680 = "2182A_1_ch1"
                    # "measure 2182A 1 channel 1 (2182A_1_ch1)"
                    n1369 = local read "2182A 1 addr"() -> (w1685:u8)
                    n1370 = Number To Decimal String(number=w1685) -> (decimal integer string=w1686:string)  [unwired: 1 in]
                    n1371 = GPIB Clear(3:w1686) -> ()  [unwired: 1 in, 2 out]
                    n1372 = Build Array (concatenate)(w1681, w1680) -> (w1679:string[])
                    n1373 = Concatenate Strings(w1684, w1680, "\t") -> (w1683:string)
                  }
                }
                n1374 = property on="Figure_axis" class="Arr (strict)"("Value"=w1672) -> ()  [unwired: 2 in, 2 out]
                n1375 = property on="data_caption" class="Str"("Value"=w1674) -> ()  [unwired: 2 in, 2 out]
              }
              frame #17 {
